vi "Format Fit Output.vi"(5 "Fit Model":T4, 7 "f(x,a)":T1, 8 "Error In":errorcluster, 9 "Fit Results":T2, 10 "Additional Data":variant, 11 "Data in":T3) -> (0 "Error Out":errorcluster, 1 "Fit Parameters Uncertainties Cluster":variant, 3 "Fit Parameters Cluster":variant)   [LabVIEW 2019]
uses:
  Fit Models.ctl
  <vilib>/gmath/NumericalOptimization/LM model function reference.ctl
  <vilib>/Utility/error.llb/DialogType.ctl
  Gaussian/Gaussian Fit Results v2.ctl
  Asymmetric Gaussian/Asymmetric Gaussian Fit Results v2.ctl
  Lorentzian/Lorentzian Fit Results v2.ctl
  Asymmetric Lorentzian/Asymmetric Lorentzian Fit Results v2.ctl
  Gaussian-Lorentzian/Gaussian-Lorentzian Fit Results v2.ctl
  Lorentzian-Gaussian/Lorentzian-Gaussian Fit Results v2.ctl
  D-Only Fixed Parameters.ctl
  Two Connected Gaussians/Two H-Connected Gaussians Fit Parameters.ctl
  Two Connected Gaussians/Two T-Connected Gaussians Fit Parameters.ctl
  Two Connected Asymmetric Gaussians/Two H-Connected Asymmetric Gaussians Fit Parameters.ctl
  Two Connected Asymmetric Gaussians/Two T-Connected Asymmetric Gaussians Fit Parameters.ctl
  Single Exponential/Single Exponential Fit Parameters v2.ctl
  IRF(X)PSED/IRF(X)PSED Fit Parameters.ctl
  IRF(X)PSED/IRF(X)PSED Fixed Parameters v3.ctl
  IRF(X)PSED/IRF(X)PSED Extraction Options.ctl
  IRF(X)PSED/Fourier Series Smoothing Option.ctl
  IRF(X)PSED/Fourier Series Truncation.ctl
  Double Exponential/Double Exponential Fit Parameters v2.ctl
  ACF-CCF/2D ACF/2D Gaussian ACF Fit Results.ctl
  ACF-CCF/2D ACF/2D Gaussian + Blinking ACF Fit Results.ctl
  ACF-CCF/2D ACF/2D Gaussian + Flow ACF Fit Results.ctl
  ACF-CCF/3D ACF/3D Gaussian ACF Fit Results.ctl
  ACF-CCF/3D ACF/3D Gaussian + Blinking ACF Fit Results.ctl
  ACF-CCF/2D ACF/2D Gaussian ACF & 2D Gaussian ACF + Flow Fit Results.ctl
  <vilib>/Analysis/NI_AALPro.lvlib
  <vilib>/gmath/NI_Gmath.lvlib
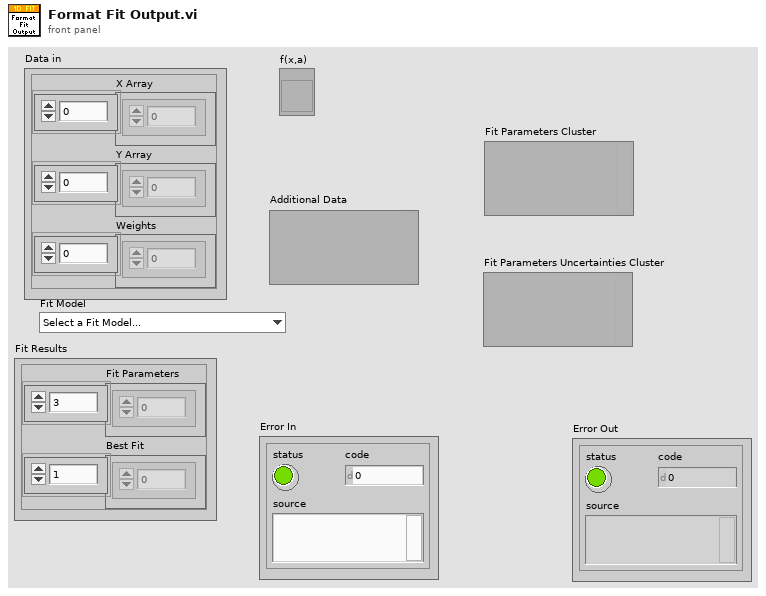
[diagram p1: front panel]
types:
  T1 = typedef "NI_Gmath.lvlib/LM model function reference.ctl" = refnum<vi>
  T2 = cluster{"Fit Parameters":dbl[], "Best Fit":dbl[]}
  T3 = cluster{"X Array":dbl[], "Y Array":dbl[], "Weights":dbl[]}
  T4 = typedef "Fit Models.ctl" = enum16{"Select a Fit Model...", "           Single Peak", "Gaussian", "Asymmetric Gaussian", "Lorentzian", "Asymmetric Lorentzian", "Gaussian/Lorentzian", "Lorentzian/Gaussian", "           Double Peak", "Two Gaussians", "Two Asymmetric Gaussians", "Two H-Connected Gaussians", "Two T-Connected Gaussians", "Two H-Connected Asymmetric Gaussians", "Two T-Connected Asymmetric Gaussians", "           Triple Peak", "Three Gaussians", "Three Asymmetric Gaussians", "              Decays", "1-Exponential", "IRF*PSED", "2-Exponentials", "               ACF", "2D Gaussian ACF", "2D Gaussian + Blinking ACF", "2D Gaussian + Flow ACF", "3D Gaussian ACF", "3D Gaussian + Blinking ACF", "             Multiplot", "2D Gaussian ACF & 2D Gaussian + Flow ACF"}
  T5 = typedef "D-Only Fixed Parameters.ctl" = cluster{"Fix D-only Peak Location":bool, "Peak Location":dbl, "Fix D-only Peak FWHM":bool, "Peak FWHM":dbl}
  T6 = typedef "IRF(X)PSED Fixed Parameters v3.ctl" = cluster{"order":i32, "T":dbl, "Time Constant Array":dbl[], "{S_k, C_k, phi_k, e_k} arrays":cluster{"S_k Array":dbl[], "C_k Array":dbl[], "phi_k Array":dbl[], "e_k Array":dbl[]}, "IRF Extraction Options":T7}
  T7 = typedef "IRF(X)PSED Extraction Options.ctl" = cluster{"Time Constant for IRF Extraction":dbl[unit], "IRF Order":i32, "Fourier Series Smoothing":T8, "Noise Threshold":dbl, "Smoothing Width":dbl, "Fourier Series Truncation":T9, "Truncation Order":i32, "Save Power Spectrum":bool}
  T8 = typedef "Fourier Series Smoothing Option.ctl" = enum16{"None", "Lanczos Factors", "Fejer Summation"}
  T9 = typedef "Fourier Series Truncation.ctl" = enum16{"Automatic", "Fixed"}
  T10 = typedef "DialogType.ctl" = u16
  T11 = typedef "Gaussian Fit Results v2.ctl" = cluster{"Amplitude":dbl, "Peak":dbl, "SDV":dbl, "FWHM":dbl, "Integral":dbl, "RMSE":dbl, "R^2":dbl}
  T12 = typedef "Asymmetric Gaussian Fit Results v2.ctl" = cluster{"Amplitude":dbl, "Peak":dbl, "SDV-":dbl, "SDV+":dbl, "Mean":dbl, "SDV":dbl, "FWHM":dbl, "Integral":dbl, "RMSE":dbl, "R^2":dbl}
  T13 = typedef "Lorentzian Fit Results v2.ctl" = cluster{"Amplitude":dbl, "Peak":dbl, "FWHM":dbl, "Integral":dbl, "RMSE":dbl, "R^2":dbl}
  T14 = typedef "Asymmetric Lorentzian Fit Results v2.ctl" = cluster{"Amplitude":dbl, "Peak":dbl, "FWHM-":dbl, "FWHM+":dbl, "Integral":dbl, "RMSE":dbl, "R^2":dbl}
  T15 = typedef "Gaussian-Lorentzian Fit Results v2.ctl" = cluster{"Amplitude":dbl, "Peak":dbl, "SDV-":dbl, "FWHM+":dbl, "Mean":dbl, "FWHM":dbl, "Integral":dbl, " RMSE":dbl, "R^2":dbl}
  T16 = typedef "Lorentzian-Gaussian Fit Results v2.ctl" = cluster{"Amplitude":dbl, "Peak":dbl, "FWHM-":dbl, "SDV+":dbl, "Mean":dbl, "FWHM":dbl, "Integral":dbl, "RMSE":dbl, "R^2":dbl}
  T17 = typedef "Two H-Connected Gaussians Fit Parameters.ctl" = cluster{"Gaussian Parameters":T11[], "Bridge Amplitude ":dbl}
  T18 = typedef "Two T-Connected Gaussians Fit Parameters.ctl" = cluster{"Gaussian Parameters":T11[], "Bridge Amplitude ":dbl, "Bridge Slope":dbl}
  T19 = typedef "Two H-Connected Asymmetric Gaussians Fit Parameters.ctl" = cluster{"Asymmetric Gaussian Parameters":T12[], "Bridge Amplitude":dbl}
  T20 = typedef "Two T-Connected Asymmetric Gaussians Fit Parameters.ctl" = cluster{"Asymmetric Gaussian Parameters":T12[], "Bridge Amplitude":dbl, "Bridge Slope":dbl}
  T21 = typedef "Single Exponential Fit Parameters v2.ctl" = cluster{"Amplitude":dbl, "Time Constant":dbl, "Baseline":dbl, "Mean":dbl, "SDV":dbl, "FWHM":dbl, "Integral":dbl, "MSE":dbl, "R^2":dbl}
  T22 = typedef "IRF(X)PSED Fit Parameters.ctl" = cluster{"Offset":dbl, "Amplitudes":dbl[], "Time Constants":dbl[], "Baseline":dbl, "Lifetime":dbl, "IRF order":dbl, "Period":dbl, "SDV":dbl, "FWHM":dbl, "Integral":dbl, "MSE":dbl, "R^2":dbl}
  T23 = typedef "Double Exponential Fit Parameters v2.ctl" = cluster{"A1":dbl, "tau1":dbl, "A2":dbl, "tau2":dbl, "Baseline":dbl, "Mean":dbl, "SDV":dbl, "Integral":dbl, "MSE":dbl, "R^2":dbl}
  T24 = typedef "2D Gaussian ACF Fit Results.ctl" = cluster{"Amplitude":dbl, "Diffusion Time":dbl, "RMSE":dbl, "R^2":dbl}
  T25 = typedef "2D Gaussian + Blinking ACF Fit Results.ctl" = cluster{"Amplitude":dbl, "Diffusion Time":dbl, "Blinking Fraction":dbl, "Blinking Time Constant":dbl, "RMSE":dbl, "R^2":dbl}
  T26 = typedef "2D Gaussian + Flow ACF Fit Results.ctl" = cluster{"Amplitude":dbl, "Diffusion Time":dbl, "Translation Time":dbl, "RMSE":dbl, "R^2":dbl}
  T27 = typedef "3D Gaussian ACF Fit Results.ctl" = cluster{"Amplitude":dbl, "Diffusion Time":dbl, "Aspect Ratio":dbl, "RMSE":dbl, "R^2":dbl}
  T28 = typedef "3D Gaussian + Blinking ACF Fit Results.ctl" = cluster{"Amplitude":dbl, "Diffusion Time":dbl, "Aspect Ratio":dbl, "Blinking Fraction":dbl, "Blinking Time Constant":dbl, "RMSE":dbl, "R^2":dbl}
  T29 = typedef "2D Gaussian ACF & 2D Gaussian ACF + Flow Fit Results.ctl" = cluster{"Amplitude 1":dbl, "Diffusion Time":dbl, "Amplitude 2":dbl, "Translation Time":dbl, "RMSE":dbl, "R^2":dbl}
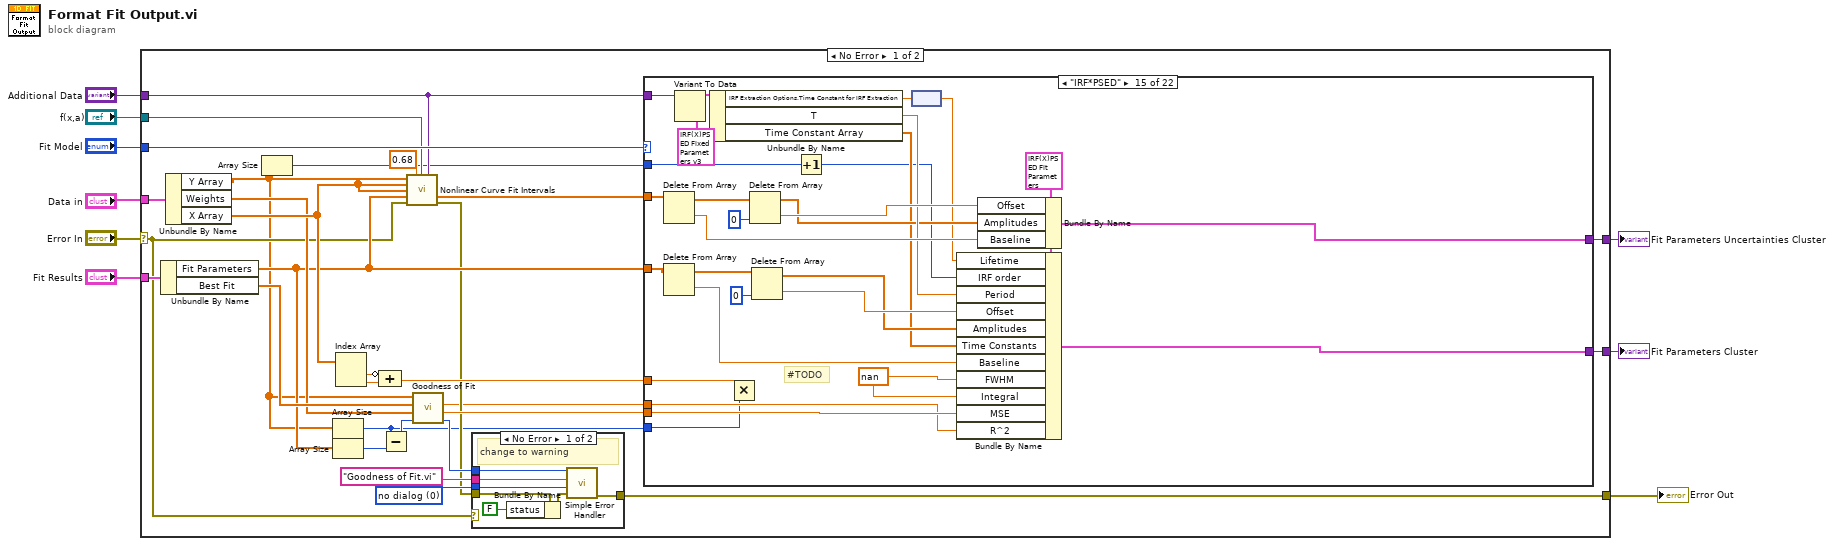
[diagram p0: block diagram]
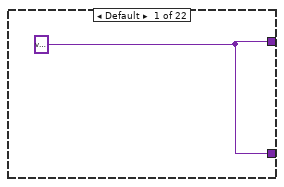
[diagram p3: hidden frame]
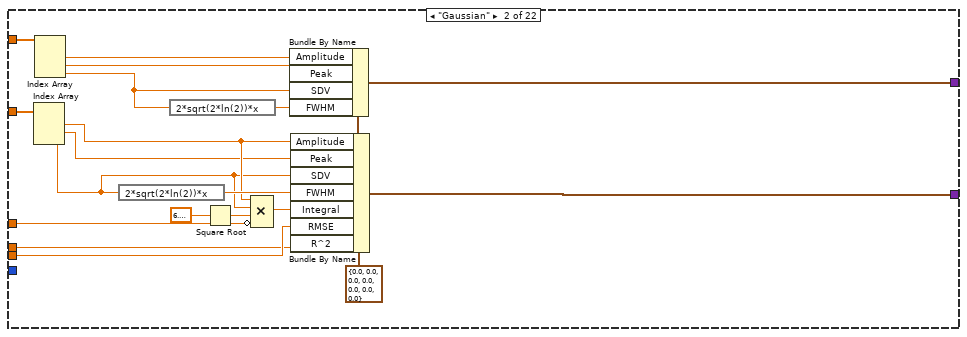
[diagram p4: hidden frame]
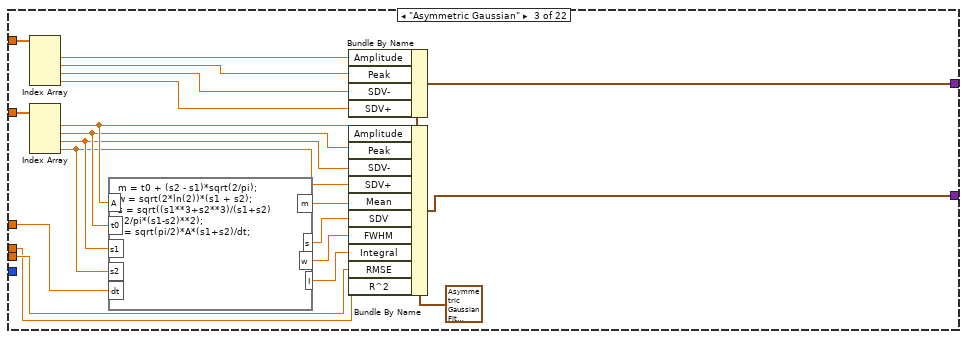
[diagram p5: hidden frame]
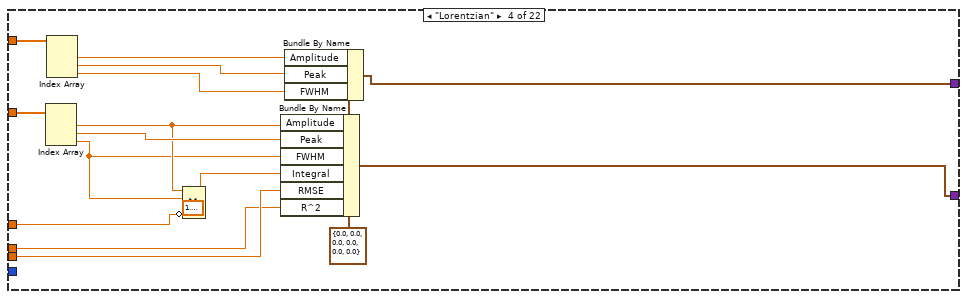
[diagram p6: hidden frame]
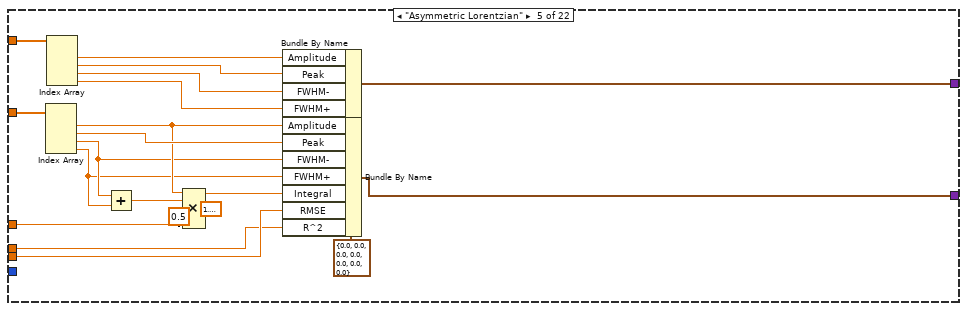
[diagram p7: hidden frame]
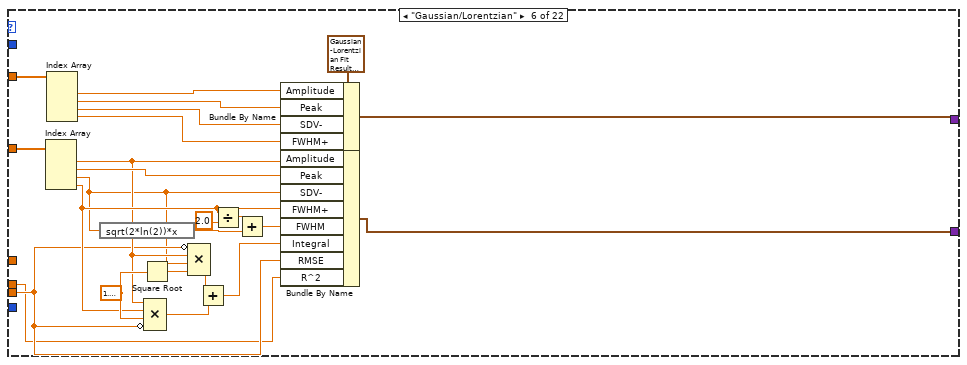
[diagram p8: hidden frame]
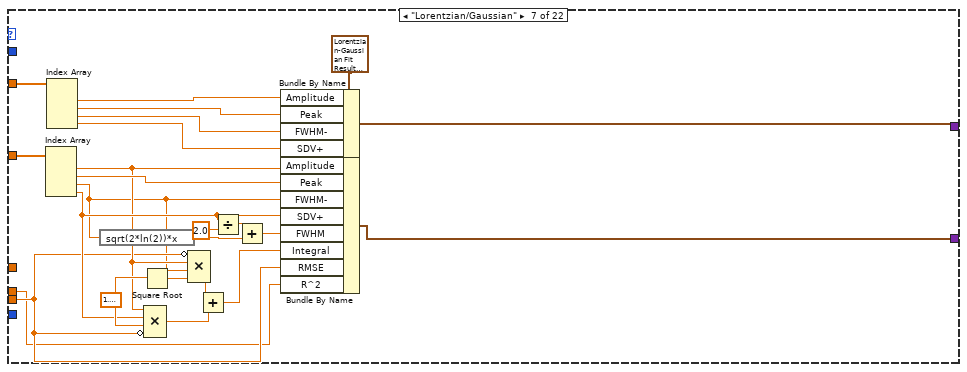
[diagram p9: hidden frame]
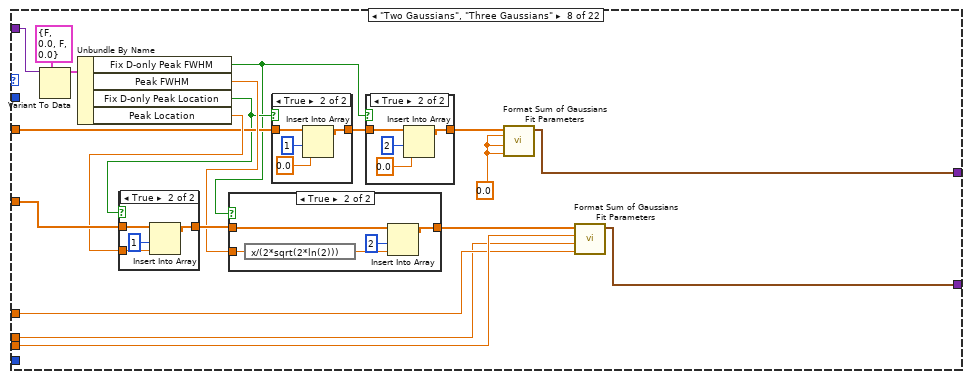
[diagram p10: hidden frame]
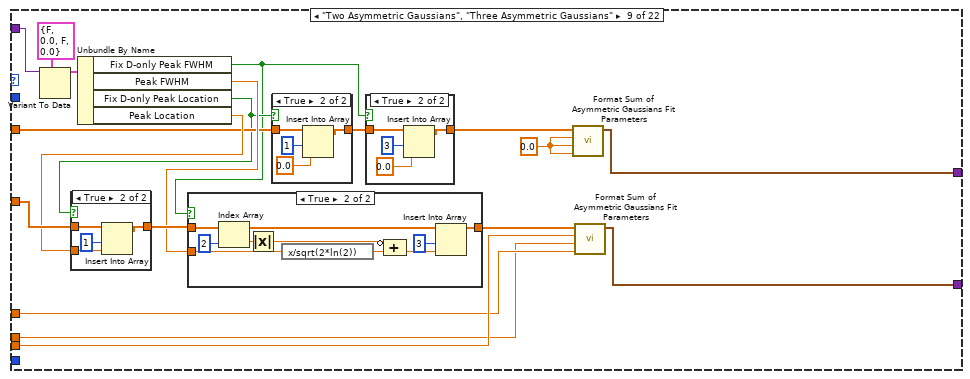
[diagram p15: hidden frame]
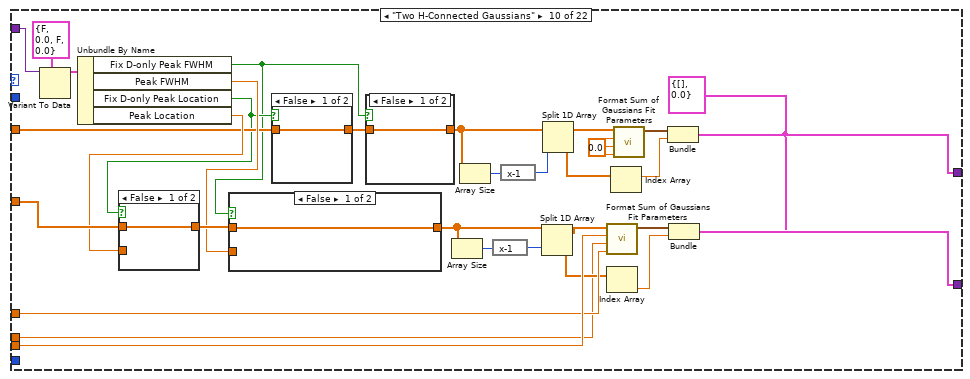
[diagram p20: hidden frame]
diagram:
  n1 = case shown="No Error" "Error In" {
    selector: "Error In" -> [w12 w635]
    tunnel: [w38 _] -> w9
    tunnel: [w37 _] -> w8
    tunnel: "Data in" -> [w30 _]
    tunnel: "Fit Results" -> [w29 _]
    tunnel: "Fit Model" -> [w27 _]
    tunnel: "f(x,a)" -> [w22 _]
    tunnel: [w17 w635] -> w2
    tunnel: "Additional Data" -> [w15 _]
    frame No Error {
      w19 = T10 0 items=["no dialog", "OK message", "continue or stop message", "OK message + warnings", "continue/stop + warnings"] ("type of dialog (OK msg:1)")
      n2 = Unbundle By Name(w29) -> ("Fit Parameters"=w24:dbl[], "Best Fit"=w28:dbl[])
      n3 = Unbundle By Name(w30) -> ("Y Array"=w11:dbl[], "Weights"=w25:dbl[], "X Array"=w26:dbl[])
      n4 = Array Size(array=w11) -> (size(s)=w10:i32)
      n5 = Array Size(array=w11) -> (size(s)=w13:i32)
      n6 = Array Size(array=w24) -> (size(s)=w33:i32)
      n7 = Index Array(array=w26) -> (element #1=w34:dbl, element #2=w36:dbl)  [unwired: 2 in]
      n8 = Compound Arithmetic op=ADD(invert w34, w36) -> (w35:dbl)
      n9 = Subtract(x=w13, y=w33) -> (x-y=w32:i32)
      n10 = call <vilib>:"Nonlinear Curve Fit Intervals.vi"("Y"=w11, "confidence level"=0.68, "f(x,a)"=w22, "data"=w15, "X"=w26, "Weight"=w26, "best fit parameters"=w24, "error in (no error)"=w12) -> ("delta best fit parameters"=w23:dbl[], "error out"=w18:errorcluster)  [unwired: 4 in, 2 out]
      n11 = call <vilib>:"Goodness of Fit.vi"("degree of freedom"=w32, "Weight"=w25, "Best Fit"=w28, "Y"=w11) -> ("error"=w21:i32, "RMSE"=w31:dbl, "R-square"=w14:dbl)  [unwired: 4 in, 1 out]
      n12 = case shown="No Error" w12 {
        selector: w12 -> [_ w46]
        tunnel: w21 -> [w45 _]
        tunnel: "Goodness of Fit.vi" ("error source (\" \")") -> [w44 _]
        tunnel: w19 -> [w43 _]
        tunnel: w18 -> [w42 _]
        tunnel: [w41 w46] -> w17
        frame No Error {
          # "change to warning"
          n13 = Bundle By Name(cluster=w42, "status"=FALSE) -> (w40:errorcluster)
          n14 = call <vilib>:"Simple Error Handler.vi"("error code (no error:0)"=w45, "error source (\" \")"=w44, "type of dialog (OK msg:1)"=w43, "error in (no error)"=w40) -> ("error out"=w41:errorcluster)  [unwired: 1 in, 4 out]
        }
        frame Error {
        }
      }
      n15 = case shown="\"IRF*PSED\"" w27 {
        tunnel: [w47 w54 w80 w88 w112 w140 w164 w174 w214 w272 w327 w380 w439 w487 w525 w544 w557 w572 w585 w600 w617 w632] -> w38
        tunnel: [w47 w53 w79 w100 w111 w139 w163 w173 w213 w273 w328 w381 w440 w486 w524 w536 w556 w571 w584 w599 w616 w631] -> w37
        tunnel: w35 -> [_ w57 w69 w95 w117 _ _ w176 w216 w274 w329 w382 w441 w481 w522 w542 _ _ _ _ _ _]
        tunnel: w31 -> [_ w56 w78 w101 w121 w125 w150 w177 w217 w275 w330 w383 w442 w490 w526 w538 w559 w574 w587 w602 w619 w634]
        tunnel: w24 -> [_ w55 w86 w102 w122 w146 w170 w186 w226 w283 w338 w391 w450 w494 w515 w543 w558 w573 w586 w601 w618 w633]
        tunnel: w23 -> [_ w52 w85 w93 w116 w144 w168 w182 w222 w279 w334 w387 w446 w497 w520 w549 w555 w570 w583 w598 w615 w630]
        tunnel: w15 -> [_ _ _ _ _ _ _ w188 w228 w285 w340 w393 w452 _ w509 _ _ _ _ _ _ _]
        tunnel: w14 -> [_ w48 w67 w87 w103 w123 w147 w172 w211 w256 w308 w363 w421 w484 w523 w531 w553 w568 w581 w597 w613 w628]
        tunnel: w13 -> [_ _ _ _ _ _ _ _ _ _ _ _ _ w480 w521 w529 _ _ _ _ _ _]
        tunnel: w10 -> [_ _ _ _ _ _ _ _ _ _ _ _ _ _ w500 _ _ _ _ _ _ _]
        frame Default {
          w47 = variant
        }
        frame "Gaussian" {
          w65 = T11 {"Amplitude"=0.0, "Peak"=0.0, "SDV"=0.0, "FWHM"=0.0, "Integral"=0.0, "RMSE"=0.0, "R^2"=0.0} ("Gaussian Fit Parameters")
          n16 = Index Array(array=w55) -> (element #1=w60:dbl, element #2=w59:dbl, element #3=w58:dbl)  [unwired: 3 in]
          n17 = Index Array(array=w52) -> (element #1=w51:dbl, element #2=w50:dbl, element #3=w49:dbl)  [unwired: 3 in]
          n18 = expression code="2*sqrt(2*ln(2))*x"(w58) -> (w64:dbl)
          n19 = expression code="2*sqrt(2*ln(2))*x"(w49) -> (w66:dbl)
          n20 = Square Root(x=6.283185307179586) -> (sqrt(x)=w62:dbl)
          n21 = Compound Arithmetic op=MULTIPLY(w60, w58, w62, invert w57) -> (w63:dbl)
          n22 = Bundle By Name(cluster=w65, "Amplitude"=w51, "Peak"=w50, "SDV"=w49, "FWHM"=w66) -> (w54:T11)
          n23 = Bundle By Name(cluster=w65, "Amplitude"=w60, "Peak"=w59, "SDV"=w58, "FWHM"=w64, "Integral"=w63, "RMSE"=w56, "R^2"=w48) -> (w53:T11)
        }
        frame "Asymmetric Gaussian" {
          w84 = T12 {"Amplitude"=0.0, "Peak"=0.0, "SDV-"=0.0, "SDV+"=0.0, "Mean"=0.0, "SDV"=0.0, "FWHM"=0.0, "Integral"=0.0, "RMSE"=0.0, "R^2"=0.0} ("Lorentz Fit Parameters")
          n24 = Index Array(array=w85) -> (element #1=w83:dbl, element #2=w82:dbl, element #3=w81:dbl, element #4=w68:dbl)  [unwired: 4 in]
          n25 = Index Array(array=w86) -> (element #1=w73:dbl, element #2=w72:dbl, element #3=w71:dbl, element #4=w70:dbl)  [unwired: 4 in]
          n26 = formula code="m = t0 + (s2 - s1)*sqrt(2/pi);\nw = sqrt(2*ln(2))*(s1 + s2);\ns = sqrt((s1**3+s2**3)/(s1+s2)\n- 2/pi*(s1-s2)**2);\nI = sqrt(pi/2)*A*(s1+s2)/dt;"("t0"=w72, "s1"=w71, "s2"=w70, "A"=w73, "dt"=w69) -> ("m"=w74:dbl, "w"=w76:dbl, "s"=w75:dbl, "I"=w77:dbl)
          n27 = Bundle By Name(cluster=w84, "Amplitude"=w83, "Peak"=w82, "SDV-"=w81, "SDV+"=w68) -> (w80:T12)
          n28 = Bundle By Name(cluster=w84, "Amplitude"=w73, "Peak"=w72, "SDV-"=w71, "SDV+"=w70, "Mean"=w74, "SDV"=w75, "FWHM"=w76, "Integral"=w77, "RMSE"=w78, "R^2"=w67) -> (w79:T12)
        }
        frame "Lorentzian" {
          w92 = T13 {"Amplitude"=0.0, "Peak"=0.0, "FWHM"=0.0, "Integral"=0.0, "RMSE"=0.0, "R^2"=0.0} ("Lorentz Fit Parameters")
          n29 = Index Array(array=w102) -> (element #1=w98:dbl, element #2=w99:dbl, element #3=w97:dbl)  [unwired: 3 in]
          n30 = Index Array(array=w93) -> (element #1=w91:dbl, element #2=w90:dbl, element #3=w89:dbl)  [unwired: 3 in]
          n31 = Compound Arithmetic op=MULTIPLY(w98, w97, 1.5707963267948966, invert w95) -> (w94:dbl)
          n32 = Bundle By Name(cluster=w92, "Amplitude"=w98, "Peak"=w99, "FWHM"=w97, "Integral"=w94, "RMSE"=w101, "R^2"=w87) -> (w100:T13)
          n33 = Bundle By Name(cluster=w92, "Amplitude"=w91, "Peak"=w90, "FWHM"=w89) -> (w88:T13)
        }
        frame "Asymmetric Lorentzian" {
          w110 = T14 {"Amplitude"=0.0, "Peak"=0.0, "FWHM-"=0.0, "FWHM+"=0.0, "Integral"=0.0, "RMSE"=0.0, "R^2"=0.0} ("Asymmetric Lorentz Fit Parameters")
          n34 = Index Array(array=w122) -> (element #1=w119:dbl, element #2=w120:dbl, element #3=w108:dbl, element #4=w107:dbl)  [unwired: 4 in]
          n35 = Index Array(array=w116) -> (element #1=w115:dbl, element #2=w114:dbl, element #3=w113:dbl, element #4=w109:dbl)  [unwired: 4 in]
          n36 = Add(x=w108, y=w107) -> (x+y=w106:dbl)
          n37 = Compound Arithmetic op=MULTIPLY(w119, w106, 1.5707963267948966, 0.5 ("value"), invert w117) -> (w104:dbl)
          n38 = Bundle By Name(cluster=w110, "Amplitude"=w115, "Peak"=w114, "FWHM-"=w113, "FWHM+"=w109) -> (w112:T14)
          n39 = Bundle By Name(cluster=w110, "Amplitude"=w119, "Peak"=w120, "FWHM-"=w108, "FWHM+"=w107, "Integral"=w104, "RMSE"=w121, "R^2"=w103) -> (w111:T14)
        }
        frame "Gaussian/Lorentzian" {
          w135 = 1.5707963267948966
          w138 = T15 {"Amplitude"=0.0, "Peak"=0.0, "SDV-"=0.0, "FWHM+"=0.0, "Mean"=0.0, "FWHM"=0.0, "Integral"=0.0, " RMSE"=0.0, "R^2"=0.0} ("Gaussian/Lorentzian Fit Parameters")
          n40 = Index Array(array=w146) -> (element #1=w126:dbl, element #2=w145:dbl, element #3=w124:dbl, element #4=w127:dbl)  [unwired: 4 in]
          n41 = Index Array(array=w144) -> (element #1=w143:dbl, element #2=w142:dbl, element #3=w141:dbl, element #4=w137:dbl)  [unwired: 4 in]
          n42 = expression code="sqrt(2*ln(2))*x"(w124) -> (w130:dbl)
          n43 = Square Root(x=w135) -> (sqrt(x)=w136:dbl)
          n44 = Compound Arithmetic op=MULTIPLY(w126, w127, w135, invert w125) -> (w134:dbl)
          n45 = Compound Arithmetic op=MULTIPLY(invert w125, w126, w124, w136) -> (w133:dbl)
          n46 = Add(x=w133, y=w134) -> (x+y=w128:dbl)
          n47 = Divide(x=w127, y=2.0) -> (x/y=w132:dbl)
          n48 = Add(x=w132, y=w130) -> (x+y=w129:dbl)
          n49 = Bundle By Name(cluster=w138, "Amplitude"=w143, "Peak"=w142, "SDV-"=w141, "FWHM+"=w137) -> (w140:T15)
          n50 = Bundle By Name(cluster=w138, "Amplitude"=w126, "Peak"=w145, "SDV-"=w124, "FWHM+"=w127, "FWHM"=w129, "Integral"=w128, "RMSE"=w125, "R^2"=w123) -> (w139:T15)
        }
        frame "Lorentzian/Gaussian" {
          w148 = T16 {"Amplitude"=0.0, "Peak"=0.0, "FWHM-"=0.0, "SDV+"=0.0, "Mean"=0.0, "FWHM"=0.0, "Integral"=0.0, "RMSE"=0.0, "R^2"=0.0} ("Lorentzian/Gaussian Fit Parameters")
          w160 = 1.5707963267948966
          n51 = Index Array(array=w170) -> (element #1=w151:dbl, element #2=w169:dbl, element #3=w149:dbl, element #4=w152:dbl)  [unwired: 4 in]
          n52 = Index Array(array=w168) -> (element #1=w167:dbl, element #2=w166:dbl, element #3=w165:dbl, element #4=w162:dbl)  [unwired: 4 in]
          n53 = expression code="sqrt(2*ln(2))*x"(w149) -> (w155:dbl)
          n54 = Square Root(x=w160) -> (sqrt(x)=w161:dbl)
          n55 = Compound Arithmetic op=MULTIPLY(w151, w152, w160, invert w150) -> (w159:dbl)
          n56 = Compound Arithmetic op=MULTIPLY(invert w150, w151, w149, w161) -> (w158:dbl)
          n57 = Add(x=w158, y=w159) -> (x+y=w153:dbl)
          n58 = Divide(x=w152, y=2.0) -> (x/y=w157:dbl)
          n59 = Add(x=w157, y=w155) -> (x+y=w154:dbl)
          n60 = Bundle By Name(cluster=w148, "Amplitude"=w167, "Peak"=w166, "FWHM-"=w165, "SDV+"=w162) -> (w164:T16)
          n61 = Bundle By Name(cluster=w148, "Amplitude"=w151, "Peak"=w169, "FWHM-"=w149, "SDV+"=w152, "FWHM"=w154, "Integral"=w153, "RMSE"=w150, "R^2"=w147) -> (w163:T16)
        }
        frame "Two Gaussians", "Three Gaussians" {
          w171 = 0.0 ("MSE")
          n62 = Variant To Data(type=T5 {"Fix D-only Peak Location"=FALSE, "Peak Location"=0.0, "Fix D-only Peak FWHM"=FALSE, "Peak FWHM"=0.0} ("Fixed Parameters"), Variant=w188) -> (data=w187:T5)  [unwired: 1 in, 1 out]
          n63 = Unbundle By Name(w187) -> ("Fix D-only Peak FWHM"=w179:bool, "Peak FWHM"=w183:dbl, "Fix D-only Peak Location"=w181:bool, "Peak Location"=w184:dbl)
          n64 = case shown="True" w181 {
            tunnel: w186 -> [w206 w210]
            tunnel: [w206 w209] -> w185
            tunnel: w184 -> [_ w207]
            frame False {
            }
            frame True {
              n65 = Insert Into Array(array=w210, index=1 ("length"), new element=w207) -> (w209:dbl[])
            }
          }
          n66 = case shown="True" w179 {
            tunnel: w185 -> [w200 w205]
            tunnel: [w200 w204] -> w178
            tunnel: w183 -> [_ w202]
            frame False {
            }
            frame True {
              n67 = expression code="x/(2*sqrt(2*ln(2)))"(w202) -> (w201:dbl)
              n68 = Insert Into Array(array=w205, index=2, new element=w201) -> (w204:dbl[])
            }
          }
          n69 = case shown="True" w181 {
            tunnel: w182 -> [w195 w199]
            tunnel: [w195 w198] -> w180
            frame False {
            }
            frame True {
              n70 = Insert Into Array(array=w199, index=1 ("length"), new element=0.0 ("new element/subarray")) -> (w198:dbl[])
            }
          }
          n71 = case shown="True" w179 {
            tunnel: w180 -> [w190 w194]
            tunnel: [w190 w193] -> w175
            frame False {
            }
            frame True {
              n72 = Insert Into Array(array=w194, index=2, new element=0.0 ("new element/subarray")) -> (w193:dbl[])
            }
          }
          n73 = call "Format Sum of Gaussians Fit Parameters.vi"("Step Size"=w171, "R^2"=w171, "MSE"=w171, "Best Fit Parameters"=w175) -> ("Array of Gaussian Fit Parameters"=w174:T11[])  [unwired: 6 in, 1 out]
          n74 = call "Format Sum of Gaussians Fit Parameters.vi"("Step Size"=w176, "R^2"=w172, "MSE"=w177, "Best Fit Parameters"=w178) -> ("Array of Gaussian Fit Parameters"=w173:T11[])  [unwired: 6 in, 1 out]
        }
        frame "Two Asymmetric Gaussians", "Three Asymmetric Gaussians" {
          w212 = 0.0 ("MSE")
          n75 = Variant To Data(type=T5 {"Fix D-only Peak Location"=FALSE, "Peak Location"=0.0, "Fix D-only Peak FWHM"=FALSE, "Peak FWHM"=0.0} ("Fixed Parameters"), Variant=w228) -> (data=w227:T5)  [unwired: 1 in, 1 out]
          n76 = Unbundle By Name(w227) -> ("Fix D-only Peak FWHM"=w219:bool, "Peak FWHM"=w223:dbl, "Fix D-only Peak Location"=w221:bool, "Peak Location"=w224:dbl)
          n77 = case shown="True" w221 {
            tunnel: w226 -> [w250 w254]
            tunnel: [w250 w253] -> w225
            tunnel: w224 -> [_ w251]
            frame False {
            }
            frame True {
              n78 = Insert Into Array(array=w254, index=1 ("length"), new element=w251) -> (w253:dbl[])
            }
          }
          n79 = case shown="True" w219 {
            tunnel: w225 -> [w240 w245]
            tunnel: [w240 w249] -> w218
            tunnel: w223 -> [_ w247]
            frame False {
            }
            frame True {
              n80 = Index Array(array=w245, index=2) -> (element=w242:dbl)
              n81 = Absolute Value(x=w242) -> (abs(x)=w241:dbl)
              n82 = expression code="x/sqrt(2*ln(2))"(w247) -> (w246:dbl)
              n83 = Compound Arithmetic op=ADD(invert w241, w246) -> (w243:dbl)
              n84 = Insert Into Array(array=w245, index=3, new element=w243) -> (w249:dbl[])
            }
          }
          n85 = case shown="True" w221 {
            tunnel: w222 -> [w235 w239]
            tunnel: [w235 w238] -> w220
            frame False {
            }
            frame True {
              n86 = Insert Into Array(array=w239, index=1 ("length"), new element=0.0 ("new element/subarray")) -> (w238:dbl[])
            }
          }
          n87 = case shown="True" w219 {
            tunnel: w220 -> [w230 w234]
            tunnel: [w230 w233] -> w215
            frame False {
            }
            frame True {
              n88 = Insert Into Array(array=w234, index=3, new element=0.0 ("new element/subarray")) -> (w233:dbl[])
            }
          }
          n89 = call "Format Sum of Asymmetric Gaussians Fit Parameters.vi"("Step Size"=w212, "R^2"=w212, "MSE"=w212, "Best Fit Parameters"=w215) -> ("Array of Asymmetric Gaussian Fit Parameters"=w214:T12[])  [unwired: 6 in, 1 out]
          n90 = call "Format Sum of Asymmetric Gaussians Fit Parameters.vi"("Step Size"=w216, "R^2"=w211, "MSE"=w217, "Best Fit Parameters"=w218) -> ("Array of Asymmetric Gaussian Fit Parameters"=w213:T12[])  [unwired: 6 in, 1 out]
        }
        frame "Two H-Connected Gaussians" {
          w259 = T17 {"Gaussian Parameters"=[], "Bridge Amplitude "=0.0} ("Bridged Gaussians Parameters")
          w255 = 0.0 ("MSE")
          n91 = Variant To Data(type=T5 {"Fix D-only Peak Location"=FALSE, "Peak Location"=0.0, "Fix D-only Peak FWHM"=FALSE, "Peak FWHM"=0.0} ("Fixed Parameters"), Variant=w285) -> (data=w284:T5)  [unwired: 1 in, 1 out]
          n92 = Unbundle By Name(w284) -> ("Fix D-only Peak FWHM"=w276:bool, "Peak FWHM"=w280:dbl, "Fix D-only Peak Location"=w278:bool, "Peak Location"=w281:dbl)
          n93 = case shown="False" w278 {
            tunnel: w283 -> [w303 w307]
            tunnel: [w303 w306] -> w282
            tunnel: w281 -> [_ w304]
            frame False {
            }
            frame True {
              n94 = Insert Into Array(array=w307, index=1 ("length"), new element=w304) -> (w306:dbl[])
            }
          }
          n95 = case shown="False" w276 {
            tunnel: w282 -> [w297 w302]
            tunnel: [w297 w301] -> w266
            tunnel: w280 -> [_ w299]
            frame False {
            }
            frame True {
              n96 = expression code="x/(2*sqrt(2*ln(2)))"(w299) -> (w298:dbl)
              n97 = Insert Into Array(array=w302, index=2, new element=w298) -> (w301:dbl[])
            }
          }
          n98 = case shown="False" w278 {
            tunnel: w279 -> [w292 w296]
            tunnel: [w292 w295] -> w277
            frame False {
            }
            frame True {
              n99 = Insert Into Array(array=w296, index=1 ("length"), new element=0.0 ("new element/subarray")) -> (w295:dbl[])
            }
          }
          n100 = case shown="False" w276 {
            tunnel: w277 -> [w287 w291]
            tunnel: [w287 w290] -> w270
            frame False {
            }
            frame True {
              n101 = Insert Into Array(array=w291, index=2, new element=0.0 ("new element/subarray")) -> (w290:dbl[])
            }
          }
          n102 = Array Size(array=w266) -> (size(s)=w267:i32)
          n103 = Array Size(array=w270) -> (size(s)=w269:i32)
          n104 = expression code="x-1"(w267) -> (w265:i32)
          n105 = expression code="x-1"(w269) -> (w268:i32)
          n106 = Split 1D Array(array=w266, index=w265) -> (first subarray=w264:dbl[], second subarray=w258:dbl[])
          n107 = Split 1D Array(array=w270, index=w268) -> (first subarray=w271:dbl[], second subarray=w262:dbl[])
          n108 = call "Format Sum of Gaussians Fit Parameters.vi"("Step Size"=w274, "R^2"=w256, "MSE"=w275, "Best Fit Parameters"=w264) -> ("Array of Gaussian Fit Parameters"=w260:T11[])  [unwired: 6 in, 1 out]
          n109 = Index Array(array=w258) -> (element=w257:dbl)  [unwired: 1 in]
          n110 = Index Array(array=w262) -> (element=w261:dbl)  [unwired: 1 in]
          n111 = call "Format Sum of Gaussians Fit Parameters.vi"("Step Size"=w255, "R^2"=w255, "MSE"=w255, "Best Fit Parameters"=w271) -> ("Array of Gaussian Fit Parameters"=w263:T11[])  [unwired: 6 in, 1 out]
          n112 = Bundle(cluster=w259, "Gaussian Parameters"=w263, "Bridge Amplitude"=w261) -> (w272:T17)
          n113 = Bundle(cluster=w259, "Gaussian Parameters"=w260, "Bridge Amplitude"=w257) -> (w273:T17)
        }
        frame "Two T-Connected Gaussians" {
          w314 = T18 {"Gaussian Parameters"=[], "Bridge Amplitude "=0.0, "Bridge Slope"=0.0} ("Bridged Gaussians Parameters")
          w309 = 0.0 ("MSE")
          n114 = Variant To Data(type=T5 {"Fix D-only Peak Location"=FALSE, "Peak Location"=0.0, "Fix D-only Peak FWHM"=FALSE, "Peak FWHM"=0.0} ("Fixed Parameters"), Variant=w340) -> (data=w339:T5)  [unwired: 1 in, 1 out]
          n115 = Unbundle By Name(w339) -> ("Fix D-only Peak FWHM"=w331:bool, "Peak FWHM"=w335:dbl, "Fix D-only Peak Location"=w333:bool, "Peak Location"=w336:dbl)
          n116 = case shown="True" w333 {
            tunnel: w338 -> [w358 w362]
            tunnel: [w358 w361] -> w337
            tunnel: w336 -> [_ w359]
            frame False {
            }
            frame True {
              n117 = Insert Into Array(array=w362, index=1 ("length"), new element=w359) -> (w361:dbl[])
            }
          }
          n118 = case shown="True" w331 {
            tunnel: w337 -> [w352 w357]
            tunnel: [w352 w356] -> w321
            tunnel: w335 -> [_ w354]
            frame False {
            }
            frame True {
              n119 = expression code="x/(2*sqrt(2*ln(2)))"(w354) -> (w353:dbl)
              n120 = Insert Into Array(array=w357, index=2, new element=w353) -> (w356:dbl[])
            }
          }
          n121 = case shown="True" w333 {
            tunnel: w334 -> [w347 w351]
            tunnel: [w347 w350] -> w332
            frame False {
            }
            frame True {
              n122 = Insert Into Array(array=w351, index=1 ("length"), new element=0.0 ("new element/subarray")) -> (w350:dbl[])
            }
          }
          n123 = case shown="True" w331 {
            tunnel: w332 -> [w342 w346]
            tunnel: [w342 w345] -> w325
            frame False {
            }
            frame True {
              n124 = Insert Into Array(array=w346, index=2, new element=0.0 ("new element/subarray")) -> (w345:dbl[])
            }
          }
          n125 = Array Size(array=w321) -> (size(s)=w322:i32)
          n126 = Array Size(array=w325) -> (size(s)=w324:i32)
          n127 = expression code="x-2"(w322) -> (w320:i32)
          n128 = expression code="x-2"(w324) -> (w323:i32)
          n129 = Split 1D Array(array=w321, index=w320) -> (first subarray=w319:dbl[], second subarray=w313:dbl[])
          n130 = Split 1D Array(array=w325, index=w323) -> (first subarray=w326:dbl[], second subarray=w317:dbl[])
          n131 = call "Format Sum of Gaussians Fit Parameters.vi"("Step Size"=w329, "R^2"=w308, "MSE"=w330, "Best Fit Parameters"=w319) -> ("Array of Gaussian Fit Parameters"=w315:T11[])  [unwired: 6 in, 1 out]
          n132 = Index Array(array=w313) -> (element #1=w312:dbl, element #2=w310:dbl)  [unwired: 2 in]
          n133 = Index Array(array=w317) -> (element #1=w316:dbl, element #2=w311:dbl)  [unwired: 2 in]
          n134 = call "Format Sum of Gaussians Fit Parameters.vi"("Step Size"=w309, "R^2"=w309, "MSE"=w309, "Best Fit Parameters"=w326) -> ("Array of Gaussian Fit Parameters"=w318:T11[])  [unwired: 6 in, 1 out]
          n135 = Bundle By Name(cluster=w314, "Gaussian Parameters"=w318, "Bridge Amplitude"=w316, "Bridge Slope"=w311) -> (w327:T18)
          n136 = Bundle By Name(cluster=w314, "Gaussian Parameters"=w315, "Bridge Amplitude"=w312, "Bridge Slope"=w310) -> (w328:T18)
        }
        frame "Two H-Connected Asymmetric Gaussians" {
          w371 = T19 {"Asymmetric Gaussian Parameters"=[], "Bridge Amplitude"=0.0} ("output cluster")
          w364 = 0.0 ("MSE")
          n137 = Variant To Data(type=T5 {"Fix D-only Peak Location"=FALSE, "Peak Location"=0.0, "Fix D-only Peak FWHM"=FALSE, "Peak FWHM"=0.0} ("Fixed Parameters"), Variant=w393) -> (data=w392:T5)  [unwired: 1 in, 1 out]
          n138 = Unbundle By Name(w392) -> ("Fix D-only Peak FWHM"=w384:bool, "Peak FWHM"=w388:dbl, "Fix D-only Peak Location"=w386:bool, "Peak Location"=w389:dbl)
          n139 = case shown="True" w386 {
            tunnel: w391 -> [w415 w419]
            tunnel: [w415 w418] -> w390
            tunnel: w389 -> [_ w416]
            frame False {
            }
            frame True {
              n140 = Insert Into Array(array=w419, index=1 ("length"), new element=w416) -> (w418:dbl[])
            }
          }
          n141 = case shown="True" w384 {
            tunnel: w390 -> [w405 w410]
            tunnel: [w405 w414] -> w367
            tunnel: w388 -> [_ w412]
            frame False {
            }
            frame True {
              n142 = Index Array(array=w410, index=2) -> (element=w407:dbl)
              n143 = Absolute Value(x=w407) -> (abs(x)=w406:dbl)
              n144 = expression code="x/sqrt(2*ln(2))"(w412) -> (w411:dbl)
              n145 = Compound Arithmetic op=ADD(invert w406, w411) -> (w408:dbl)
              n146 = Insert Into Array(array=w410, index=3, new element=w408) -> (w414:dbl[])
            }
          }
          n147 = case shown="True" w386 {
            tunnel: w387 -> [w400 w404]
            tunnel: [w400 w403] -> w385
            frame False {
            }
            frame True {
              n148 = Insert Into Array(array=w404, index=1 ("length"), new element=0.0 ("new element/subarray")) -> (w403:dbl[])
            }
          }
          n149 = case shown="True" w384 {
            tunnel: w385 -> [w395 w399]
            tunnel: [w395 w398] -> w377
            frame False {
            }
            frame True {
              n150 = Insert Into Array(array=w399, index=3, new element=0.0 ("new element/subarray")) -> (w398:dbl[])
            }
          }
          n151 = Array Size(array=w377) -> (size(s)=w379:i32)
          n152 = Array Size(array=w367) -> (size(s)=w369:i32)
          n153 = expression code="x-1"(w379) -> (w378:i32)
          n154 = expression code="x-1"(w369) -> (w370:i32)
          n155 = Split 1D Array(array=w377, index=w378) -> (first subarray=w376:dbl[], second subarray=w374:dbl[])
          n156 = Split 1D Array(array=w367, index=w370) -> (first subarray=w368:dbl[], second subarray=w366:dbl[])
          n157 = call "Format Sum of Asymmetric Gaussians Fit Parameters.vi"("Step Size"=w364, "R^2"=w364, "MSE"=w364, "Best Fit Parameters"=w376) -> ("Array of Asymmetric Gaussian Fit Parameters"=w375:T12[])  [unwired: 6 in, 1 out]
          n158 = Index Array(array=w374) -> (element=w373:dbl)  [unwired: 1 in]
          n159 = call "Format Sum of Asymmetric Gaussians Fit Parameters.vi"("Step Size"=w382, "R^2"=w363, "MSE"=w383, "Best Fit Parameters"=w368) -> ("Array of Asymmetric Gaussian Fit Parameters"=w372:T12[])  [unwired: 6 in, 1 out]
          n160 = Index Array(array=w366) -> (element=w365:dbl)  [unwired: 1 in]
          n161 = Bundle(cluster=w371, "Asymmetric Gaussian Parameters"=w375, "Bridge Amplitude"=w373) -> (w380:T19)
          n162 = Bundle(cluster=w371, "Asymmetric Gaussian Parameters"=w372, "Bridge Amplitude"=w365) -> (w381:T19)
        }
        frame "Two T-Connected Asymmetric Gaussians" {
          w422 = T20 {"Asymmetric Gaussian Parameters"=[], "Bridge Amplitude"=0.0, "Bridge Slope"=0.0} ("Two T-Connected Asymmetric Gaussian Parameters")
          w420 = 0.0 ("MSE")
          n163 = Variant To Data(type=T5 {"Fix D-only Peak Location"=FALSE, "Peak Location"=0.0, "Fix D-only Peak FWHM"=FALSE, "Peak FWHM"=0.0} ("Fixed Parameters"), Variant=w452) -> (data=w451:T5)  [unwired: 1 in, 1 out]
          n164 = Unbundle By Name(w451) -> ("Fix D-only Peak FWHM"=w443:bool, "Peak FWHM"=w447:dbl, "Fix D-only Peak Location"=w445:bool, "Peak Location"=w448:dbl)
          n165 = case shown="True" w445 {
            tunnel: w450 -> [w474 w478]
            tunnel: [w474 w477] -> w449
            tunnel: w448 -> [_ w475]
            frame False {
            }
            frame True {
              n166 = Insert Into Array(array=w478, index=1 ("length"), new element=w475) -> (w477:dbl[])
            }
          }
          n167 = case shown="True" w443 {
            tunnel: w449 -> [w464 w469]
            tunnel: [w464 w473] -> w427
            tunnel: w447 -> [_ w471]
            frame False {
            }
            frame True {
              n168 = Index Array(array=w469, index=2) -> (element=w466:dbl)
              n169 = Absolute Value(x=w466) -> (abs(x)=w465:dbl)
              n170 = expression code="x/sqrt(2*ln(2))"(w471) -> (w470:dbl)
              n171 = Compound Arithmetic op=ADD(invert w465, w470) -> (w467:dbl)
              n172 = Insert Into Array(array=w469, index=3, new element=w467) -> (w473:dbl[])
            }
          }
          n173 = case shown="True" w445 {
            tunnel: w446 -> [w459 w463]
            tunnel: [w459 w462] -> w444
            frame False {
            }
            frame True {
              n174 = Insert Into Array(array=w463, index=1 ("length"), new element=0.0 ("new element/subarray")) -> (w462:dbl[])
            }
          }
          n175 = case shown="True" w443 {
            tunnel: w444 -> [w454 w458]
            tunnel: [w454 w457] -> w436
            frame False {
            }
            frame True {
              n176 = Insert Into Array(array=w458, index=3, new element=0.0 ("new element/subarray")) -> (w457:dbl[])
            }
          }
          n177 = Array Size(array=w436) -> (size(s)=w438:i32)
          n178 = Array Size(array=w427) -> (size(s)=w429:i32)
          n179 = expression code="x-2"(w438) -> (w437:i32)
          n180 = expression code="x-2"(w429) -> (w430:i32)
          n181 = Split 1D Array(array=w436, index=w437) -> (first subarray=w435:dbl[], second subarray=w433:dbl[])
          n182 = Split 1D Array(array=w427, index=w430) -> (first subarray=w428:dbl[], second subarray=w426:dbl[])
          n183 = call "Format Sum of Asymmetric Gaussians Fit Parameters.vi"("Step Size"=w420, "R^2"=w420, "MSE"=w420, "Best Fit Parameters"=w435) -> ("Array of Asymmetric Gaussian Fit Parameters"=w434:T12[])  [unwired: 6 in, 1 out]
          n184 = Index Array(array=w433) -> (element #1=w432:dbl, element #2=w424:dbl)  [unwired: 2 in]
          n185 = call "Format Sum of Asymmetric Gaussians Fit Parameters.vi"("Step Size"=w441, "R^2"=w421, "MSE"=w442, "Best Fit Parameters"=w428) -> ("Array of Asymmetric Gaussian Fit Parameters"=w431:T12[])  [unwired: 6 in, 1 out]
          n186 = Index Array(array=w426) -> (element #1=w425:dbl, element #2=w423:dbl)  [unwired: 2 in]
          n187 = Bundle By Name(cluster=w422, "Asymmetric Gaussian Parameters"=w434, "Bridge Amplitude"=w432, "Bridge Slope"=w424) -> (w439:T20)
          n188 = Bundle By Name(cluster=w422, "Asymmetric Gaussian Parameters"=w431, "Bridge Amplitude"=w425, "Bridge Slope"=w423) -> (w440:T20)
        }
        frame "1-Exponential" {
          w498 = T21 {"Amplitude"=0.0, "Time Constant"=0.0, "Baseline"=0.0, "Mean"=0.0, "SDV"=0.0, "FWHM"=0.0, "Integral"=0.0, "MSE"=0.0, "R^2"=0.0} ("Single Exponential Fit Parameters")
          n189 = Index Array(array=w494) -> (element #1=w489:dbl, element #2=w492:dbl, element #3=w483:dbl)  [unwired: 3 in]
          n190 = Index Array(array=w497) -> (element #1=w496:dbl, element #2=w495:dbl, element #3=w485:dbl)  [unwired: 3 in]
          n191 = Compound Arithmetic op=MULTIPLY(w489, w492, invert w481) -> (w488:dbl)
          n192 = Multiply(x=w481, y=w480) -> (x*y=w479:dbl)
          n193 = Compound Arithmetic op=ADD(w488, w479) -> (w482:dbl)
          n194 = Multiply(x=w492, y=0.6931471805599453) -> (x*y=w491:dbl)
          n195 = Bundle By Name(cluster=w498, "Amplitude"=w496, "Time Constant"=w495, "Baseline"=w485) -> (w487:T21)
          n196 = Bundle By Name(cluster=w498, "Amplitude"=w489, "Time Constant"=w492, "Baseline"=w483, "FWHM"=w491, "Integral"=w482, "MSE"=w490, "R^2"=w484) -> (w486:T21)
        }
        frame "IRF*PSED" {
          w510 = nan ("FWHM")
          w527 = T22 {"Offset"=0.0, "Amplitudes"=[], "Time Constants"=[], "Baseline"=0.0, "Lifetime"=0.0, "IRF order"=0.0, "Period"=0.0, "SDV"=0.0, "FWHM"=0.0, "Integral"=0.0, "MSE"=0.0, "R^2"=0.0} ("IRF*PSED Fit Parameters")
          # "#TODO"
          n197 = Delete From Array(array=w520) -> (deleted portion=w519:dbl, array with subset deleted=w518:dbl[])  [unwired: 2 in]
          n198 = Delete From Array(array=w515) -> (deleted portion=w514:dbl, array with subset deleted=w512:dbl[])  [unwired: 2 in]
          n199 = Variant To Data(type=T6 {"order"=0, "T"=0.0, "Time Constant Array"=[], "{S_k, C_k, phi_k, e_k} arrays"={"S_k Array"=[], "C_k Array"=[], "phi_k Array"=[], "e_k Array"=[]}, "IRF Extraction Options"={"Time Constant for IRF Extraction"=1e-18, "IRF Order"=0, "Fourier Series Smoothing"=enum."None", "Noise Threshold"=0.0, "Smoothing Width"=0.0, "Fourier Series Truncation"=enum."Automatic", "Truncation Order"=0, "Save Power Spectrum"=FALSE}} ("IRF*PSED fixed Parameters"), Variant=w509) -> (data=w507:T6)  [unwired: 1 in, 1 out]
          n200 = Unbundle By Name(w507) -> ("IRF Extraction Options.Time Constant for IRF Extraction"=w506:dbl[unit], "T"=w505:dbl, "Time Constant Array"=w502:dbl[])
          n201 = Multiply(x=w522, y=w521) -> ()  [unwired: 1 out]
          n202 = Delete From Array(array=w518, index=0) -> (deleted portion=w516:dbl, array with subset deleted=w504:dbl[])  [unwired: 1 in]
          n203 = Delete From Array(array=w512, index=0) -> (deleted portion=w511:dbl, array with subset deleted=w503:dbl[])  [unwired: 1 in]
          n204 = Increment(x=w500) -> (x+1=w499:i32)
          n205 = node(w506) -> (w501:dbl)
          n206 = Bundle By Name(cluster=w527, "Lifetime"=w501, "IRF order"=w499, "Period"=w505, "Offset"=w511, "Amplitudes"=w503, "Time Constants"=w502, "Baseline"=w514, "FWHM"=w510, "Integral"=w510, "MSE"=w526, "R^2"=w523) -> (w524:T22)
          n207 = Bundle By Name(cluster=w527, "Offset"=w516, "Amplitudes"=w504, "Baseline"=w519) -> (w525:T22)
        }
        frame "2-Exponentials" {
          w537 = T23 {"A1"=0.0, "tau1"=0.0, "A2"=0.0, "tau2"=0.0, "Baseline"=0.0, "Mean"=0.0, "SDV"=0.0, "Integral"=0.0, "MSE"=0.0, "R^2"=0.0} ("Double Exponential Fit Parameters")
          n208 = Index Array(array=w543) -> (element #1=w535:dbl, element #2=w534:dbl, element #3=w533:dbl, element #4=w532:dbl, element #5=w528:dbl)  [unwired: 5 in]
          n209 = formula code="float64 N;\nN = A1*t1+A2*t2;\nm = (A1*t1**2+A2*t2**2)/N;\ns = 2*sqrt(A1*t1*A2*t2)*abs(t2-t1)/N;\nI = (A1*t1 + A2*t2)/dt;"("t1"=w534, "A2"=w533, "t2"=w532, "dt"=w542, "A1"=w535, "nb"=w529, "B"=w528) -> ("m"=w541:dbl, "s"=w540:dbl, "I"=w539:dbl)
          n210 = Index Array(array=w549) -> (element #1=w548:dbl, element #2=w547:dbl, element #3=w546:dbl, element #4=w545:dbl, element #5=w530:dbl)  [unwired: 5 in]
          n211 = Bundle By Name(cluster=w537, "A1"=w548, "tau1"=w547, "A2"=w546, "tau2"=w545, "Baseline"=w530) -> (w544:T23)
          n212 = Bundle By Name(cluster=w537, "A1"=w535, "tau1"=w534, "A2"=w533, "tau2"=w532, "Baseline"=w528, "Mean"=w541, "SDV"=w540, "MSE"=w538, "Integral"=w539, "R^2"=w531) -> (w536:T23)
        }
        frame "2D Gaussian ACF" {
          w560 = T24 {"Amplitude"=0.0, "Diffusion Time"=0.0, "RMSE"=0.0, "R^2"=0.0} ("2D ACF Fit Parameters")
          n213 = Index Array(array=w555) -> (element #1=w554:dbl, element #2=w552:dbl)  [unwired: 2 in]
          n214 = Index Array(array=w558) -> (element #1=w551:dbl, element #2=w550:dbl)  [unwired: 2 in]
          n215 = Bundle By Name(cluster=w560, "Amplitude"=w554, "Diffusion Time"=w552) -> (w557:T24)
          n216 = Bundle By Name(cluster=w560, "Amplitude"=w551, "Diffusion Time"=w550, "RMSE"=w559, "R^2"=w553) -> (w556:T24)
        }
        frame "2D Gaussian + Blinking ACF" {
          w575 = T25 {"Amplitude"=0.0, "Diffusion Time"=0.0, "Blinking Fraction"=0.0, "Blinking Time Constant"=0.0, "RMSE"=0.0, "R^2"=0.0} ("2D Gaussian + Blinking ACF Fit Parameters")
          n217 = Index Array(array=w573) -> (element #1=w566:dbl, element #2=w565:dbl, element #3=w562:dbl, element #4=w561:dbl)  [unwired: 4 in]
          n218 = Index Array(array=w570) -> (element #1=w569:dbl, element #2=w567:dbl, element #3=w564:dbl, element #4=w563:dbl)  [unwired: 4 in]
          n219 = Bundle By Name(cluster=w575, "Amplitude"=w569, "Diffusion Time"=w567, "Blinking Fraction"=w564, "Blinking Time Constant"=w563) -> (w572:T25)
          n220 = Bundle By Name(cluster=w575, "Amplitude"=w566, "Diffusion Time"=w565, "Blinking Fraction"=w562, "Blinking Time Constant"=w561, "RMSE"=w574, "R^2"=w568) -> (w571:T25)
        }
        frame "2D Gaussian + Flow ACF" {
          w588 = T26 {"Amplitude"=0.0, "Diffusion Time"=0.0, "Translation Time"=0.0, "RMSE"=0.0, "R^2"=0.0} ("2D Gaussian + Blinking ACF Fit Parameters")
          n221 = Index Array(array=w586) -> (element #1=w579:dbl, element #2=w578:dbl, element #3=w576:dbl)  [unwired: 3 in]
          n222 = Index Array(array=w583) -> (element #1=w582:dbl, element #2=w580:dbl, element #3=w577:dbl)  [unwired: 3 in]
          n223 = Bundle By Name(cluster=w588, "Amplitude"=w582, "Diffusion Time"=w580, "Translation Time"=w577) -> (w585:T26)
          n224 = Bundle By Name(cluster=w588, "Amplitude"=w579, "Diffusion Time"=w578, "Translation Time"=w576, "RMSE"=w587, "R^2"=w581) -> (w584:T26)
        }
        frame "3D Gaussian ACF" {
          w593 = T27 {"Amplitude"=0.0, "Diffusion Time"=0.0, "Aspect Ratio"=0.0, "RMSE"=0.0, "R^2"=0.0} ("3D ACF Fit Parameters")
          n225 = Index Array(array=w598) -> (element #1=w591:dbl, element #2=w596:dbl, element #3=w592:dbl)  [unwired: 3 in]
          n226 = Index Array(array=w601) -> (element #1=w595:dbl, element #2=w594:dbl, element #3=w590:dbl)  [unwired: 3 in]
          n227 = Absolute Value(x=w590) -> (abs(x)=w589:dbl)
          n228 = Bundle By Name(cluster=w593, "Amplitude"=w591, "Diffusion Time"=w596, "Aspect Ratio"=w592) -> (w600:T27)
          n229 = Bundle By Name(cluster=w593, "Amplitude"=w595, "Diffusion Time"=w594, "Aspect Ratio"=w589, "RMSE"=w602, "R^2"=w597) -> (w599:T27)
        }
        frame "3D Gaussian + Blinking ACF" {
          w609 = T28 {"Amplitude"=0.0, "Diffusion Time"=0.0, "Aspect Ratio"=0.0, "Blinking Fraction"=0.0, "Blinking Time Constant"=0.0, "RMSE"=0.0, "R^2"=0.0} ("2D Gaussian + Blinking ACF Fit Parameters")
          n230 = Index Array(array=w618) -> (element #1=w611:dbl, element #2=w610:dbl, element #3=w603:dbl, element #4=w604:dbl, element #5=w605:dbl)  [unwired: 5 in]
          n231 = Index Array(array=w615) -> (element #1=w614:dbl, element #2=w612:dbl, element #3=w606:dbl, element #4=w607:dbl, element #5=w608:dbl)  [unwired: 5 in]
          n232 = Bundle By Name(cluster=w609, "Amplitude"=w611, "Diffusion Time"=w610, "Aspect Ratio"=w603, "Blinking Fraction"=w604, "Blinking Time Constant"=w605, "RMSE"=w619, "R^2"=w613) -> (w616:T28)
          n233 = Bundle By Name(cluster=w609, "Amplitude"=w614, "Diffusion Time"=w612, "Aspect Ratio"=w606, "Blinking Fraction"=w607, "Blinking Time Constant"=w608) -> (w617:T28)
        }
        frame "2D Gaussian ACF & 2D Gaussian + Flow ACF" {
          w622 = T29 {"Amplitude 1"=0.0, "Diffusion Time"=0.0, "Amplitude 2"=0.0, "Translation Time"=0.0, "RMSE"=0.0, "R^2"=0.0} ("2D Gaussian ACF & ACF + Flow Fit Parameters")
          n234 = Index Array(array=w630) -> (element #1=w629:dbl, element #2=w627:dbl, element #3=w621:dbl, element #4=w624:dbl)  [unwired: 4 in]
          n235 = Index Array(array=w633) -> (element #1=w626:dbl, element #2=w625:dbl, element #3=w620:dbl, element #4=w623:dbl)  [unwired: 4 in]
          n236 = Bundle By Name(cluster=w622, "Amplitude 1"=w629, "Diffusion Time"=w627, "Amplitude 2"=w621, "Translation Time"=w624) -> (w632:T29)
          n237 = Bundle By Name(cluster=w622, "Amplitude 1"=w626, "Diffusion Time"=w625, "Amplitude 2"=w620, "Translation Time"=w623, "RMSE"=w634, "R^2"=w628) -> (w631:T29)
        }
      }
    }
    frame Error {
    }
  }
  "Fit Parameters Cluster" <- w8
  "Fit Parameters Uncertainties Cluster" <- w9
  "Error Out" <- w2
